vi "Select Ball Position.vi"(10 "Circles Data":T2(array[cluster]), 11 "Ball Data past":T1) -> (3 "Ball Data out":T1)   [LabVIEW 2012]
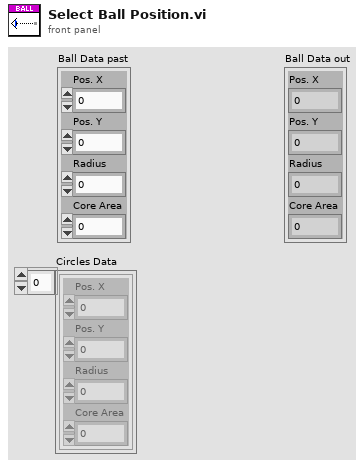
[diagram p1: front panel]
types:
  T1 = cluster{"Pos. X":i32, "Pos. Y":i32, "Radius":i32, "Core Area":i32}
  T2 = cluster{"Pos. X":i32, "Pos. Y":i32, "Radius":i32, "Core Area":i32}[]
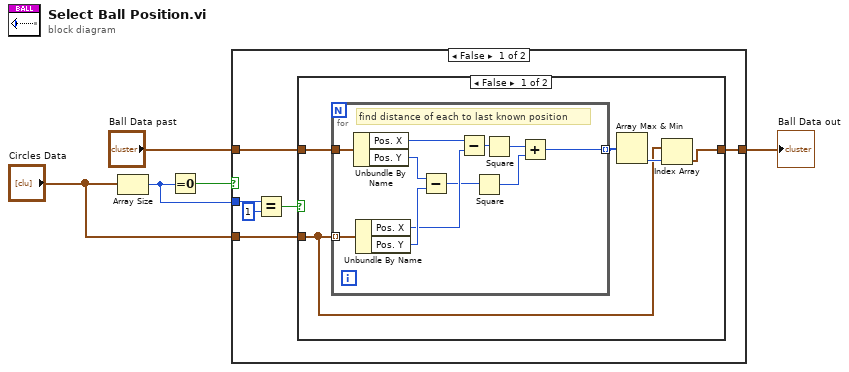
[diagram p0: block diagram]
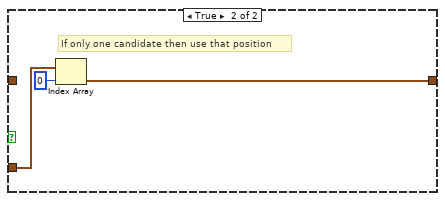
[diagram p2: hidden frame]
diagram:
  n1 = Array Size(array="Circles Data") -> (size(s)=w4:i32)
  n2 = Equal To 0?(x=w4) -> (x = 0?=w1:bool)
  n3 = case shown="False" w1 {
    tunnel: "Ball Data past" -> [w6 w31]
    tunnel: [w7 w31] -> w3
    tunnel: w4 -> [w11 _]
    tunnel: "Circles Data" -> [w8 _]
    frame False {
      n4 = Equal?(x=w11, y=1) -> (x = y?=w9:bool)
      n5 = case shown="False" w9 {
        tunnel: w8 -> [w13 w30]
        tunnel: [w12 w28] -> w7
        tunnel: w6 -> [w16 _]
        frame False {
          n6 = for {
            tunnel: w13 -> [w27] mode=indexing
            tunnel: w16 -> [w26]
            tunnel: [w17] -> w15 mode=indexing
            # "find distance of each to last known position"
            n7 = Unbundle By Name(w26) -> ("Pos. X"=w23:i32, "Pos. Y"=w25:i32)
            n8 = Unbundle By Name(w27) -> ("Pos. X"=w22:i32, "Pos. Y"=w24:i32)
            n9 = Subtract(x=w25, y=w24) -> (x-y=w21:i32)
            n10 = Subtract(x=w23, y=w22) -> (x-y=w20:i32)
            n11 = Square(x=w21) -> (x^2=w18:i32)
            n12 = Square(x=w20) -> (x^2=w19:i32)
            n13 = Add(x=w19, y=w18) -> (x+y=w17:i32)
          }
          n14 = Array Max & Min(array=w15) -> (min index (indices)=w14:i32)  [unwired: 3 out]
          n15 = Index Array(array=w13, index=w14) -> (element=w12:T1)
        }
        frame True {
          # "If only one candidate then use that position"
          n16 = Index Array(array=w30, index=0) -> (element=w28:T1)
        }
      }
    }
    frame True {
      # "If no ball found use last position"
    }
  }
  "Ball Data out" <- w3
